vi "LivePosition_Graph_CSVOut.vi"() -> ()   [LabVIEW 2015]
doc: "This program connects to the ESP301 and turns on the joystick the saves the position of each axis at a 1ms resolution. The axis positions are displayed on the VI front panel. Whenever the user says stop or the ESP301 throws an error it will stop taking data. Then you have the option of saving the times and axis positions to a csv file for later analysis. --Alex Kaufman"
uses:
  <vilib>/Native 3D Graph/xcontrol/3DPC_SurfacePlot.xctl
  <vilib>/Platform/TimedLoop/XDataNode/timing_clust.ctl
  <vilib>/Platform/TimedLoop/XDataNode/nitl_modes.ctl
  <vilib>/Platform/TimedLoop/XDataNode/wakeup.ctl
  <vilib>/Utility/file.llb/Write Delimited Spreadsheet (DBL).vi
  <vilib>/Platform/TimedLoop/XDataNode/XDataNode.xnode
  <vilib>/Platform/TimedLoop/XDataNode/XDNodeRunTimeDep.lvlib
  <userlib>/Newport ESP301/Newport ESP301.lvlib
panel:
  in  "Cancel Button":bool
  in  "OK Button":bool
  out "?":refnum<class "Base Datatype.lvclass">[](xcontrol)
  in  "?":bool
  out "Axis 3 Pos.":dbl
  out "Axis 2 Pos.":dbl
  out "Axis 1 Pos.":dbl
  # "After the graph appears press OK to accept and save the data points\nOr Press Cancel"
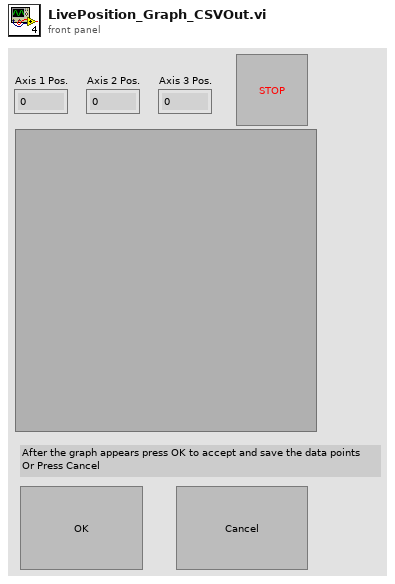
[diagram p1: front panel]
types:
  T1 = typedef "XDNodeRunTimeDep.lvlib/timing_clust.ctl" = cluster{"Expected End [f-1]":u64, "Actual End [f-1]":u64, "Finished Late? [f-1]":bool, "Expected End [i-1]":u64, "Actual End [i-1]":u64, "Finished Late? [i-1]":bool, "Expected Start [i]":u64, "Actual Start [i]":u64, "Expected Start [f]":u64, "Actual Start [f]":u64, "Source Name":string, "Structure Name":string, "Period":i64, "Deadline":i64, "Offset":i64, "Start":i64, "Priority":i32, "Timeout":i32, "Mode":T2, "Wakeup Reason":T3, "Error":errorcluster, "Source Type":string, "Secondary Source Type":string, "Global End Time":u64, "Global Start Time":u64, "Frame Duration":u64, "Iteration Duration":u64, "Assigned CPU":i32, "I/O Scan Engine Mode":u32}
  T2 = typedef "XDNodeRunTimeDep.lvlib/nitl_modes.ctl" = enum32{"No Change", "Process missed periods, maintain original phase", "Discard missed periods, maintain original phase", "Process missed periods, ignore original phase", "Discard missed periods, ignore original phase"}
  T3 = typedef "XDNodeRunTimeDep.lvlib/wakeup.ctl" = enum32{"Normal", "Aborted", "Asynchronous wakeup", "Timing source error", "Timed loop error", "Timeout"}
  T4 = typedef "NI_Matrix.lvlib/RealMatrix.ctl" = dbl[][]
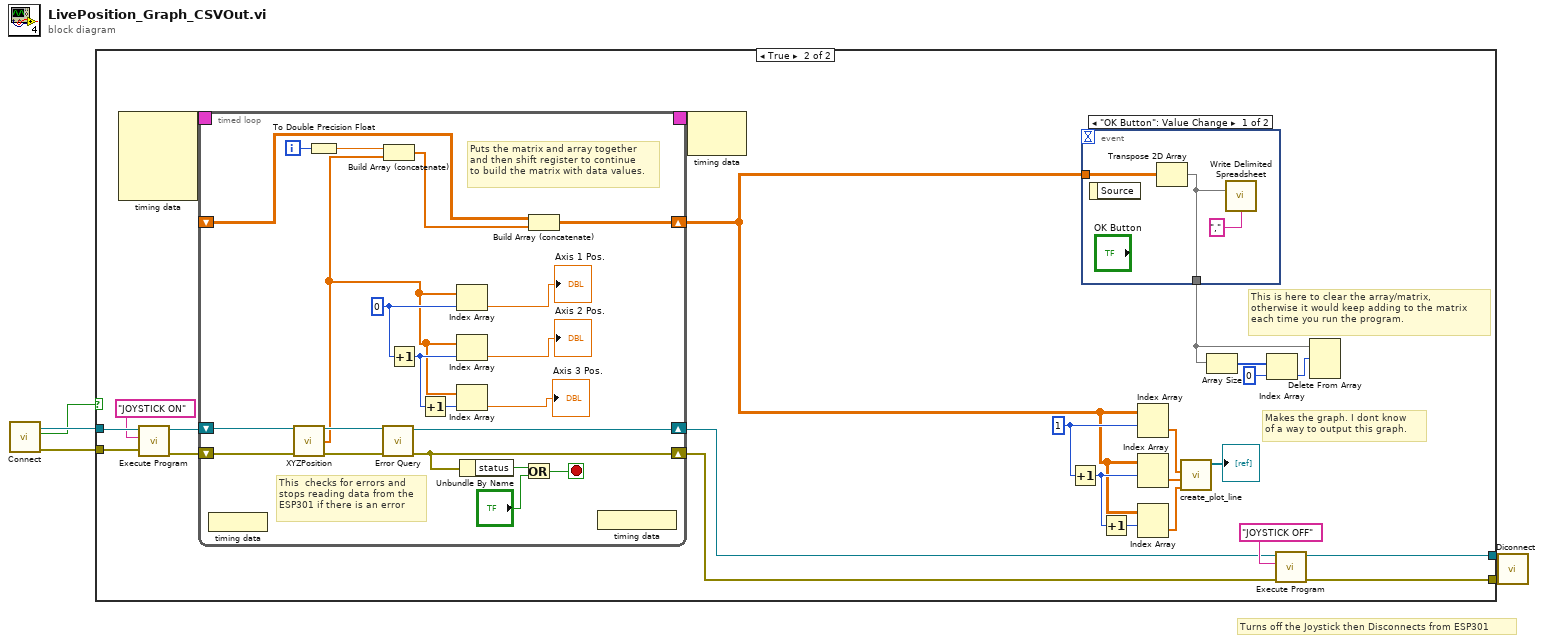
[diagram p0: block diagram]
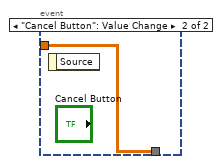
[diagram p3: hidden frame]
diagram:
  # "Turns off the Joystick then Disconnects from ESP301"
  n1 = call "Connect.vi"() -> ("error out"=w4:errorcluster, "Connected"=w3:bool, "VISA resource name out"=w5:refnum<visa-resource-name>)  [unwired: 5 in]
  n2 = case shown="True" w3 {
    tunnel: [w7 w8] -> w2
    tunnel: [w6 w9] -> w1
    tunnel: w5 -> [w7 w22]
    tunnel: w4 -> [w6 w15]
    frame False {
    }
    frame True {
      w25 = 1
      # "Makes the graph. I dont know \nof a way to output this graph."
      # "This is here to clear the array/matrix,\notherwise it would keep adding to the matrix \neach time you run the program."
      n3 = node-c288() -> (w31:T1)  [unwired: 4 in]
      n4 = call <userlib>:"Execute Program.vi"("error in (no error)"=w15, "Program Name"="JOYSTICK ON", "VISA resource name"=w22) -> ("error out"=w16:errorcluster, "VISA resource name out"=w21:refnum<visa-resource-name>)  [unwired: 3 in]
      n5 = timed-loop {
        timing: w31 -> [_]
        timing-out: [_] -> w30
        shift-right: [w52] -> w11
        shift-left: w21 -> [w56]
        shift-right: [w50] -> w10
        shift-left: w16 -> [w55]
        shift-right: [w44] -> w17
        shift-left: _ -> [w45]
        i -> [w47]
        stop <- w48 stop-if-true
        w42 = 0
        # "Puts the matrix and array together\nand then shift register to continue \nto build the matrix with data values."
        # "This  checks for errors and \nstops reading data from the\nESP301 if there is an error"
        n6 = node-c288() -> ()  [unwired: 1 in]
        n7 = call "XYZPosition.vi"("VISA resource name"=w56, "error in"=w55) -> ("VISA resource name out"=w53:refnum<visa-resource-name>, "[x,y,z]"=w39:dbl[], "error out"=w54:errorcluster)  [unwired: 11 in]
        n8 = To Double Precision Float(number=w47) -> (double precision float=w46:dbl)
        n9 = call <userlib>:"Error Query.vi"("error in (no error)"=w54, "VISA resource name"=w53) -> ("error out"=w50:errorcluster, "VISA resource name out"=w52:refnum<visa-resource-name>)  [unwired: 2 in, 2 out]
        n10 = Build Array (concatenate)(w46, w39) -> (w43:dbl[])
        n11 = Increment(x=w42) -> (x+1=w40:i32)
        n12 = Increment(x=w40) -> (x+1=w41:i32)
        n13 = Index Array(array=w39, index=w42) -> (element=→"Axis 1 Pos.":dbl)
        n14 = Index Array(array=w39, index=w40) -> (element=→"Axis 2 Pos.":dbl)
        n15 = Index Array(array=w39, index=w41) -> (element=→"Axis 3 Pos.":dbl)
        n16 = Unbundle By Name(w50) -> ("status"=w49:bool)
        n17 = Or(x=w49, y="?") -> (x .or. y?=w48:bool)
        n18 = Build Array (concatenate)(w45, w43) -> (w44:T4)
        n19 = node-c288() -> ()  [unwired: 1 out]
      }
      n20 = node-c288(w30) -> ()  [unwired: 1 out]
      n21 = Increment(x=w25) -> (x+1=w23:i32)
      n22 = event shown="[0] \"OK Button\": Value Change" {
        selector: _ -> [_ _]
        dyn-events: _ -> [_ _]
        timeout: _ -> [_ _]
        tunnel: w17 -> [w33 w35]
        tunnel: [w32 w35] -> w13
        event "OK Button": Value Change {
          n23 = event-data() -> ()  [unwired: 1 in, 1 out]
          n24 = Transpose 2D Array(2D array=w33) -> (transposed array=w32:T4)
          n25 = call-poly <vilib>:"Write Delimited Spreadsheet.vi"("2D data"=w32, "delimiter (\\t)"=",") -> ()  [unwired: 12 in, 2 out]
        }
        event "Cancel Button": Value Change {
          n26 = event-data() -> ()  [unwired: 1 in, 1 out]
        }
      }
      n27 = Increment(x=w23) -> (x+1=w24:i32)
      n28 = Index Array(array=w17, index (row)=w25) -> (element=w28:dbl[])  [unwired: 1 in]
      n29 = Index Array(array=w17, index (row)=w23) -> (element=w27:dbl[])  [unwired: 1 in]
      n30 = Index Array(array=w17, index (row)=w24) -> (element=w26:dbl[])  [unwired: 1 in]
      n31 = call <vilib>:"create_plot_line.vi"("z vector"=w26, "y vector"=w27, "x vector"=w28) -> ("plots out"=→"?":refnum<class "Base Datatype.lvclass">[])  [unwired: 2 in, 6 out]
      n32 = Array Size(array=w13) -> (size(s)=w18:i32[])
      n33 = Index Array(array=w18, index=0) -> (element=w19:i32)
      n34 = call <userlib>:"Execute Program.vi"("error in (no error)"=w10, "Program Name"="JOYSTICK OFF", "VISA resource name"=w11) -> ("error out"=w9:errorcluster, "VISA resource name out"=w8:refnum<visa-resource-name>)  [unwired: 3 in]
      n35 = Delete From Array(array=w13, length=w19) -> ()  [unwired: 2 in, 2 out]
    }
  }
  n36 = call "Diconnect.vi"("error in (no error)"=w1, "VISA resource name"=w2) -> ()  [unwired: 6 in]
